vi "Configure Frequency Sweep.vi"(0 "VISA resource name":refnum<visa-resource-name>, 1 "Enable Trigger Output (F:Disable)":bool, 2 "Enable Frequency Sweep (T:Enable)":bool=TRUE, 3 "Channel (1:Channel 1)":i32(ring)=1 items=["Channel 1"=1, "Channel 2"=2], 5 "Sweep Spacing (0: Linear)":u16(ring) items=["Linear", "Log"], 7 "Sweep Time (1.00 s)":dbl=1.0 format="%#.6g", 9 "Sweep Direction (0: Up)":u16(ring) items=["Up", "Down", "Up_Down"], 11 "error in (no error)":errorcluster, 12 "Source (0: Internal)":u16(ring) items=["Internal", "External", "Manual"], 13 "Start Frequency (100.0 Hz)":dbl=100.0 format="%#.6g", 14 "Stop Frequency  (1000.0 Hz)":dbl=1000.0 format="%#.6g") -> (4 "VISA resource name out":refnum<visa-resource-name>, 15 "error out":errorcluster)   [LabVIEW 2022 SP3, in "Siglent SDG X Series.lvlib"]
doc: "Configures and enables a frequency sweep. In the frequency sweep mode, the function generator steps from the start frequency to the stop frequency at a sweep rate.\n\nNote: Sweep function is not available for Pulse, Noise, and DC waveforms."
uses:
  Siglent SDG X Series.lvlib
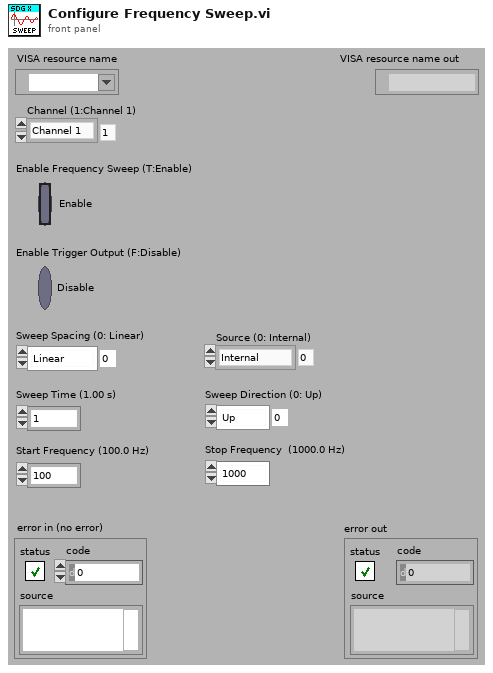
[diagram p1: front panel]
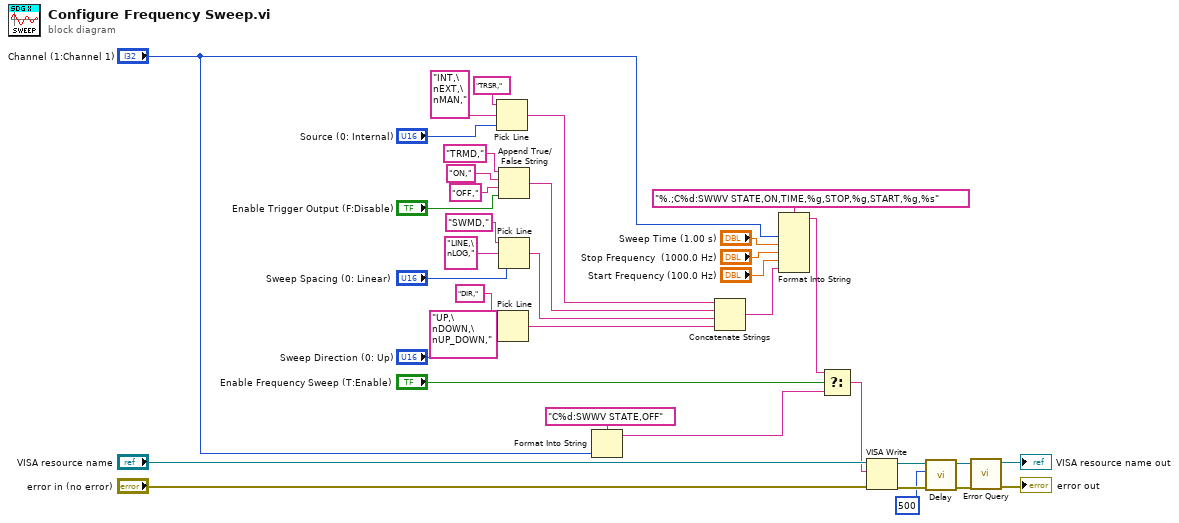
[diagram p0: block diagram]
diagram:
  n1 = Pick Line(string ("")="TRSR,", multi-line string="INT,\nEXT,\nMAN,", line index="Source (0: Internal)") -> (output string=w11:string)
  n2 = Pick Line(string ("")="DIR,", multi-line string="UP,\nDOWN,\nUP_DOWN,", line index="Sweep Direction (0: Up)") -> (output string=w14:string)
  n3 = Append True/False String(1:"Enable Trigger Output (F:Disable)", 2:"OFF,", 3:"ON,", 4:"TRMD,") -> (0:w12:string)
  n4 = Pick Line(string ("")="SWMD,", multi-line string="LINE,\nLOG,", line index="Sweep Spacing (0: Linear)") -> (output string=w13:string)
  n5 = Format Into String(format string="C%d:SWWV STATE,OFF", "Channel (1:Channel 1)") -> (resulting string=w9:string)  [unwired: 2 in, 1 out]
  n6 = Concatenate Strings(w11, w12, w13, w14) -> (w15:string)
  n7 = Format Into String(format string="%.;C%d:SWWV STATE,ON,TIME,%g,STOP,%g,START,%g,%s", "Channel (1:Channel 1)", "Sweep Time (1.00 s)", "Stop Frequency  (1000.0 Hz)", "Start Frequency (100.0 Hz)", w15) -> (resulting string=w8:string)  [unwired: 2 in, 1 out]
  n8 = Select(t=w8, s="Enable Frequency Sweep (T:Enable)", f=w9) -> (s? t:f=w7:string)
  n9 = VISA Write(VISA resource name="VISA resource name", write buffer=w7, error in (no error)="error in (no error)") -> (VISA resource name out=w3:refnum<visa-resource-name>, error out=w2:errorcluster)  [unwired: 1 out]
  n10 = call "Delay.vi"("error in (no error)"=w2, "Delay Time (10)"=u32 500, "VISA resource name"=w3) -> ("error out"=w5:errorcluster, "VISA resource name out"=w4:refnum<visa-resource-name>)  [unwired: 7 in]
  n11 = call "Error Query.vi"("error in (no error)"=w5, "VISA resource name"=w4) -> ("error out"=→"error out":errorcluster, "VISA resource name out"=→"VISA resource name out":refnum<visa-resource-name>)  [unwired: 6 in, 2 out]
